vi "rad_Apply Network Settings (Static).vi"(6 "Timeout in ms (4s)":u32=4000, 8 "error in (no error)":errorcluster, 10 "Requested settings":T1={"Hostname"="", "Serial number"="", "Product name"="", "Product code"=0, "System status"="", "Credential type"=enum."None/Unlocked", "User added?"=FALSE, "Primary NIC"={"MAC address"="", "IP Address Request Mode"=2, "IP address"="", "Subnet mask"="", "Gateway"="", "DNS server"=""}} {"Primary NIC"."IP Address Request Mode" items=["Static"=1, "DHCP/Link-Local"=2, "Link-Local Only"=4, "DHCP Only"=8]}, 11 "Existing settings":T1={"Hostname"="", "Serial number"="", "Product name"="", "Product code"=0, "System status"="", "Credential type"=enum."None/Unlocked", "User added?"=FALSE, "Primary NIC"={"MAC address"="", "IP Address Request Mode"=2, "IP address"="", "Subnet mask"="", "Gateway"="", "DNS server"=""}} {"Primary NIC"."IP Address Request Mode" items=["Static"=1, "DHCP/Link-Local"=2, "Link-Local Only"=4, "DHCP Only"=8]}) -> (0 "error out":errorcluster, 3 "Target settings out":T1={"Hostname"="", "Serial number"="", "Product name"="", "Product code"=0, "System status"="", "Credential type"=enum."None/Unlocked", "User added?"=FALSE, "Primary NIC"={"MAC address"="", "IP Address Request Mode"=2, "IP address"="", "Subnet mask"="", "Gateway"="", "DNS server"=""}} {"Primary NIC"."IP Address Request Mode" items=["Static"=1, "DHCP/Link-Local"=2, "Link-Local Only"=4, "DHCP Only"=8]})   [LabVIEW 2016]
uses:
  TypeDefs/rad_Target Information.ctl
  TypeDefs/rad_Target Network Settings.ctl
  <vilib>/nisyscfg/Save Changes (System).vi
  <vilib>/nisyscfg/Close (System).vi
  <resource>/objmgr/nisysapi.rc
  <vilib>/nisyscfg/nisyscfg.lvlib
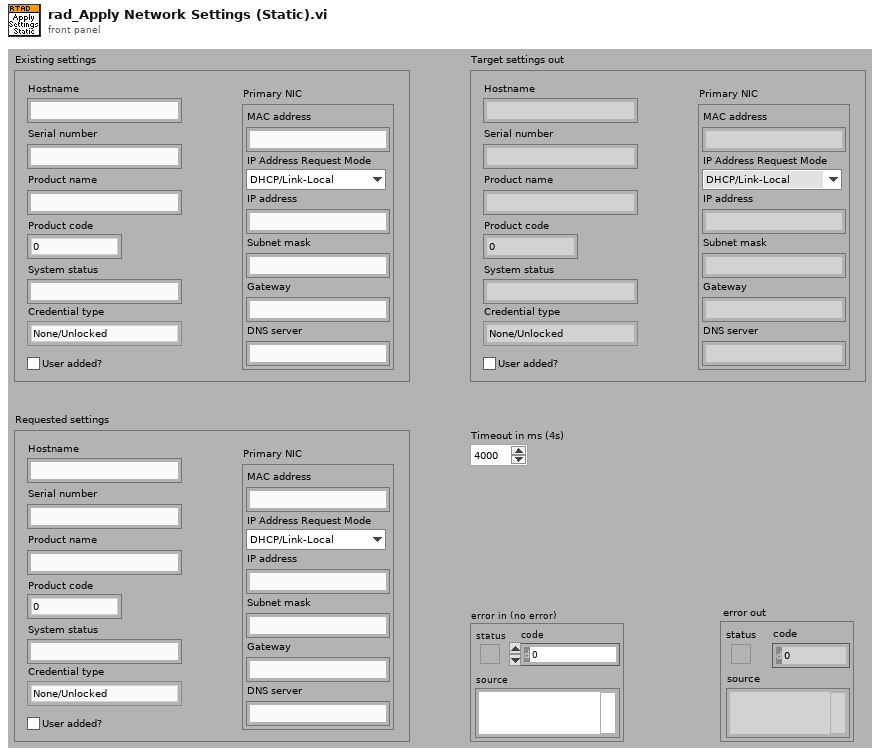
[diagram p1: front panel]
types:
  T1 = typedef "rad_Target Information.ctl" = cluster{"Hostname":string, "Serial number":string, "Product name":string, "Product code":i32, "System status":string, "Credential type":enum16{"None/Unlocked", "FTP Password", "NIAuth Credentials"}, "User added?":bool, "Primary NIC":T2}
  T2 = typedef "rad_Target Network Settings.ctl" = cluster{"MAC address":string, "IP Address Request Mode":i32, "IP address":string, "Subnet mask":string, "Gateway":string, "DNS server":string}
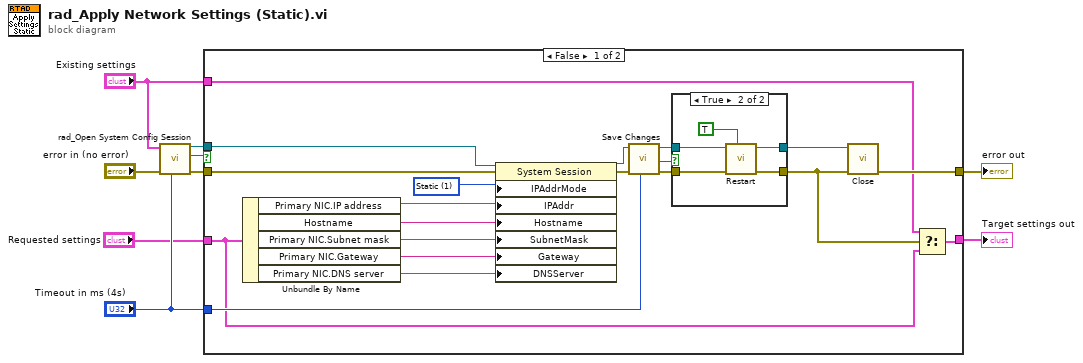
[diagram p0: block diagram]
diagram:
  n1 = call "rad_Open System Config Session.vi"("Timeout ms (4000)"="Timeout in ms (4s)", "error in (no error)"="error in (no error)", "Target settings"="Existing settings") -> ("error out"=w5:errorcluster, "Cancelled"=w4:bool, "Session out"=w7:refnum<k21>)  [unwired: 5 in, 1 out]
  n2 = case shown="False" w4 {
    tunnel: [w10 w37] -> w1
    tunnel: [w29 w38] -> w8
    tunnel: w7 -> [w28 _]
    tunnel: "Timeout in ms (4s)" -> [w27 _]
    tunnel: "Requested settings" -> [w11 _]
    tunnel: w5 -> [w14 w38]
    tunnel: "Existing settings" -> [w12 w37]
    frame False {
      w21 = 1 items=["Static"=1, "DHCP/Link-Local"=2, "Link-Local Only"=4, "DHCP Only"=8] ("Primary NIC:IP Address Request Mode")
      n3 = Unbundle By Name(w11) -> ("Primary NIC.IP address"=w26:string, "Hostname"=w25:string, "Primary NIC.Subnet mask"=w24:string, "Primary NIC.Gateway"=w23:string, "Primary NIC.DNS server"=w22:string)
      n4 = property class="System Session"(reference=w28, error in=w14, "IPAddrMode"=w21, "IPAddr"=w26, "Hostname"=w25, "SubnetMask"=w24, "Gateway"=w23, "DNSServer"=w22) -> (reference out=w20:refnum<k21>, error out=w19:errorcluster)
      n5 = call-poly <vilib>:"Save Changes.vi"("Remote Timeout (300,000 ms)"=w27, "error in (no error)"=w19, "Session in"=w20) -> ("error out"=w17:errorcluster, "Changes Require Restart"=w18:bool, "Session out"=w16:refnum<k21>)  [unwired: 5 in, 1 out]
      n6 = case shown="True" w18 {
        tunnel: w17 -> [w31 w36]
        tunnel: [w31 w35] -> w13
        tunnel: w16 -> [w30 w34]
        tunnel: [w30 w33] -> w15
        frame False {
        }
        frame True {
          n7 = call <vilib>:"Restart.vi"("Wait Until Complete (T)"=TRUE ("wait until complete (T)"), "error in (no error)"=w36, "Session in"=w34) -> ("error out"=w35:errorcluster, "Session out"=w33:refnum<k21>)  [unwired: 6 in, 1 out]
        }
      }
      n8 = call-poly <vilib>:"Close.vi"("error in (no error)"=w13, "Session in"=w15) -> ("error out"=w29:errorcluster)  [unwired: 9 in]
      n9 = Select(t=w12, s=w13, f=w11) -> (s? t:f=w10:T1)
    }
    frame True {
    }
  }
  "error out" <- w8
  "Target settings out" <- w1
